vi "G#Object_ConvertToMoreGeneric.vi"(0 "reference in":refnum<class "G#Object.lvclass">, 2 "convert to":refnum<class "G#Object.lvclass">, 5 "error in (no error)":errorcluster) -> (14 "converted reference out":refnum<class "G#Object.lvclass">, 19 "error out":errorcluster)   [LabVIEW 2017, in "G#Object.lvclass"]
doc: "Converts the input 'reference in' to the 'convert to' type specifier. This method will convert a subclass reference into a more generic parent reference including the run-time type, make the object behave like it actually belonged to the more generic class. This could be used to force a parent call from a VI that is not an overriding VI.\n\nUse this VI carefully."
uses:
  G#Object.lvclass
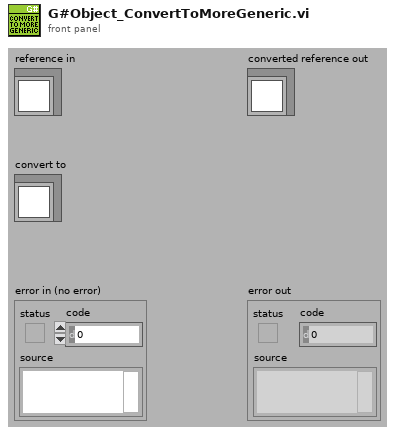
[diagram p1: front panel]
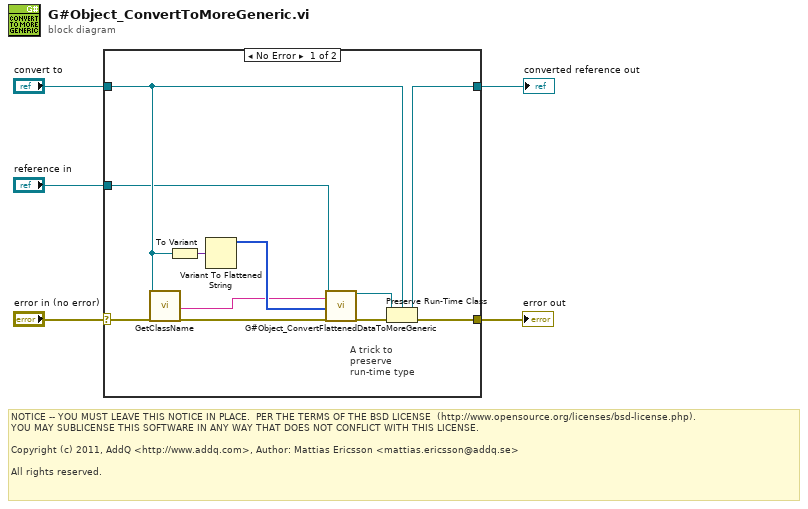
[diagram p0: block diagram]
diagram:
  # "NOTICE -- YOU MUST LEAVE THIS NOTICE IN PLACE.  PER THE TERMS OF THE BSD LICENSE  (http://www.opensource.org/licenses/bsd-license.php).\nYOU MAY SUBLICENSE THIS SOFTWARE IN ANY WAY THAT DOES NOT CONFLICT WITH THIS LICENSE.\n\nCopyright (c) 2011, AddQ <http://www.addq.com>, Author: Mattias Ericsson <mattias.ericsson@addq.se>\n\nAll rights reserved."
  n1 = case shown="No Error" "error in (no error)" {
    selector: "error in (no error)" -> [w12 w18]
    tunnel: [w16 w18] -> w4
    tunnel: "reference in" -> [w10 _]
    tunnel: [w15 w17] -> w3
    tunnel: "convert to" -> [w13 w17]
    frame No Error {
      # "A trick to\npreserve\nrun-time type"
      n2 = call-dynamic "GetClassName.vi"("reference in"=w13, "error in (no error)"=w12) -> ("full class name"=w8:string, "error out"=w11:errorcluster)  [unwired: 13 in, 3 out]
      n3 = To Variant(anything=w13) -> (Variant=w14:variant)
      n4 = Variant To Flattened String(Variant=w14) -> (1:w9:i16[])  [unwired: 1 out]
      n5 = call "G#Object_ConvertFlattenedDataToMoreGeneric.vi"("reference in"=w10, "full class name"=w8, "type string"=w9, "error in (no error)"=w11) -> ("reference converterrd"=w6:refnum<class "G#Object.lvclass">, "error out"=w7:errorcluster)  [unwired: 14 in]
      n6 = Preserve Run-Time Class(object in=w6, error in=w7, 2:w13) -> (object out=w15:refnum<class "G#Object.lvclass">, error out=w16:errorcluster)
    }
    frame Error {
    }
  }
  "error out" <- w4
  "converted reference out" <- w3
